vi "(SubVI) Get Height and Width.vi"(8 "error in (no error)":errorcluster, 11 "Refnum in":T1) -> (0 "error out":errorcluster, 1 "Height":u32, 2 "Width":u32, 3 "Refnum out":T1)   [LabVIEW 2014]
uses:
  <vilib>/userdefined/High Color/IMAQdx.ctl
  <resource>/objmgr/imaqdx.rc
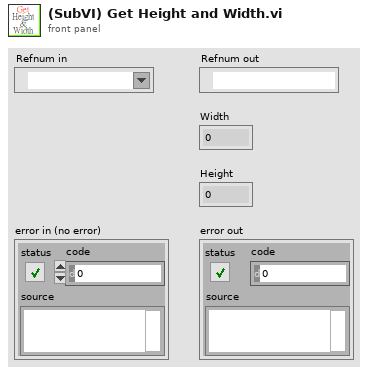
[diagram p1: front panel]
types:
  T1 = typedef "IMAQdx.ctl" = refnum<k21>
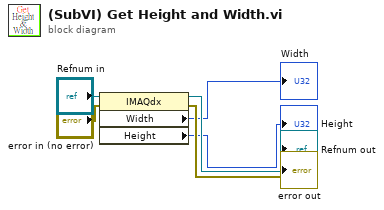
[diagram p0: block diagram]
diagram:
  n1 = property class="IMAQdx"(reference="Refnum in", error in="error in (no error)") -> (reference out=→"Refnum out":T1, error out=→"error out":errorcluster, "Width"=→"Width":u32, "Height"=→"Height":u32)
